vi "Output Complete.vi"(8 "error in  2":errorcluster, 11 "TeleOp Data Cluster 2":T1) -> (0 "error out  2":errorcluster)   [LabVIEW 2018]
uses:
  TypeDefs/Teleop Data Cluster.ctl
  TypeDefs/typedef_enum_Refnums.ctl
  <vilib>/Rock Robotics/WPI/Solenoid/WPI_SolenoidValue.ctl
  <vilib>/Rock Robotics/WPI/ThirdParty/Phoenix-LabVIEW/Motor Controller/Controls/CTRE_Phoenix_MotorControl_ControlMode.ctl
  <vilib>/Rock Robotics/WPI/Solenoid/WPI_SolenoidSetEnum.vi
  <vilib>/Rock Robotics/Network Tables/NT Write Boolean.vi
  <vilib>/Rock Robotics/Network Tables/NT Write Number.vi
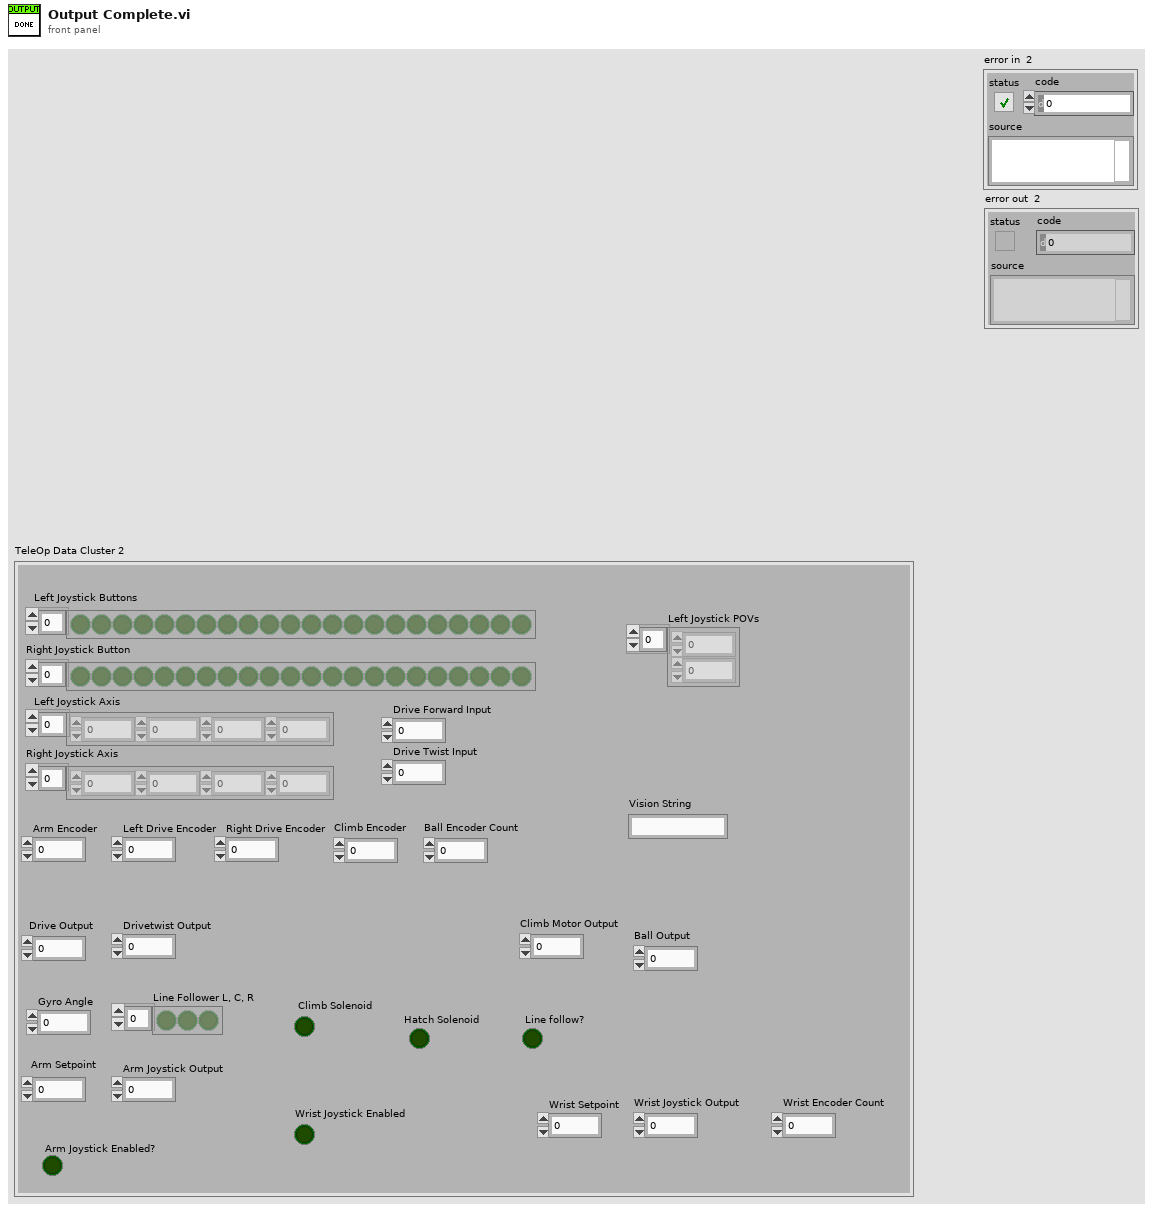
[diagram p1: front panel]
types:
  T1 = typedef "Teleop Data Cluster.ctl" = cluster{"Drive Forward Input ":dbl, "Drive Twist Input":dbl, "Drive Output":dbl, "Drivetwist Output":dbl, "Left Joystick Buttons":bool[], "Left Joystick Axis":dbl[], "Right Joystick Axis":dbl[], "Right Joystick Button":bool[], "Arm Encoder":dbl, "Left Drive Encoder":dbl, "Right Drive Encoder":dbl, "Gyro Angle ":dbl, "Arm Joystick Output  ":dbl, "Line Follower L, C, R ":bool[], "Line follow?":bool, " Climb Solenoid":bool, "Wrist Encoder Count":dbl, "Wrist Joystick Output":dbl, "Ball Encoder Count":dbl, "Ball Output":dbl, "Climb Encoder":dbl, "Climb Motor Output":dbl, " Hatch Solenoid":bool, "Arm Setpoint ":dbl, "Wrist Setpoint ":dbl, "Arm Joystick Enabled?":bool, "Wrist Joystick Enabled":bool, "Vision String":string, "Left Joystick POVs":i16[]}
  T2 = typedef "typedef_enum_Refnums.ctl" = enum16{"Ball_Encoder", "Ball_Motor", "Camera", "Linefollow_3", "Linefollow_2", "Linefollow_1", "Gyro", "Hatch_Solenoid", "Climb_Back_Solenoid", "Arm_Encoder", "Arm_Motor", "Lift_Encoder", "Drive", "Drive_Motor_R", "Drive_Motor_L", "Drive_Encoder_R", "Drive_Encoder_L", "Joy_R", "Joy_L", "Wrist_Motor", "Wrist_Encoder", "Climb Upper Limit", "Climb Lower Limit ", "Climb_Front_Motor"}
  T3 = typedef "CTRE_Phoenix_MotorControl_ControlMode.ctl" = u16
  T4 = typedef "WPI_SolenoidValue.ctl" = enum16{"Off", "On", "Forward", "Reverse"}
  T5 = typedef "WPI_SwitchDevRef.ctl" = cluster{"DevStatus":errorcluster, "DIO Channel":T6, "CntIndex":T7, "Normally Closed":bool}
  T6 = typedef "FPGA_DIOChannel.ctl" = enum8{"DIO 0", "DIO 1", "DIO 2", "DIO 3", "DIO 4", "DIO 5", "DIO 6", "DIO 7", "DIO 8", "DIO 9", "DIO MXP 0", "DIO MXP 1", "DIO MXP 2", "DIO MXP 3", "DIO MXP 4", "DIO MXP 5", "DIO MXP 6", "DIO MXP 7", "DIO MXP 8", "DIO MXP 9", "DIO MXP 10", "DIO MXP 11", "DIO MXP 12", "DIO MXP 13", "DIO MXP 14", "DIO MXP 15", "SPI Port CS1", "SPI Port CS2", "SPI Port CS3", "SPI Port MISO", "SPI Port MOSI", "Invalid"}
  T7 = typedef "FPGA_CounterCtrSystemIndex.ctl" = enum8{"Ctr 0", "Ctr 1", "Ctr 2", "Ctr 3", "Ctr 4", "Ctr 5", "Ctr 6", "Ctr 7", "Invalid"}
  T8 = typedef "WPI_MotorControlDeviceRef.ctl" = cluster{"DeviceStatus":errorcluster, "Type":T9, "PWM":cluster{"PWM Channel":T10, "DeadBand":T11}, "CAN":cluster{"Device Number":u8, "SetOutput VI Ref":variant, "GetOutput VI Ref":variant, "Enable VI Ref":variant, "Disable VI Ref":variant, "Data":variant}, "Invert":bool, "DIO PWM":cluster{"PWM \"Enable\" Channel":T10, "DIOChannel":T6, "PWM Rate":dbl}}
  T9 = typedef "WPI_MotorControlType.ctl" = enum16{"PWM", "CAN", "DIO PWM"}
  T10 = typedef "FPGA_DIOPWMChannel.ctl" = enum8{"PWM 0", "PWM 1", "PWM 2", "PWM 3", "PWM 4", "PWM 5", "PWM 6", "PWM 7", "PWM 8", "PWM 9", "PWM MXP 0", "PWM MXP 1", "PWM MXP 2", "PWM MXP 3", "PWM MXP 4", "PWM MXP 5", "PWM MXP 6", "PWM MXP 7", "PWM MXP 8", "PWM MXP 9", "Invalid"}
  T11 = typedef "WPI_PWMDeadband.ctl" = cluster{"Name":string, "maxPositivePwm":i32, "minPositivePwm":i32, "centerPwm":i32, "maxNegativePwm":i32, "minNegativePwm":i32, "angularRange":u16}
  T12 = typedef "WPI_SolenoidDevRef.ctl" = cluster{"DevStatus":errorcluster, "Pneumatics Control Module":u8, "Forward Solenoid Channel":T13, "Reverse Solenoid Channel":T13}
  T13 = typedef "WPI_SolenoidChannel.ctl" = enum8{"Solenoid 0", "Solenoid 1", "Solenoid 2", "Solenoid 3", "Solenoid 4", "Solenoid 5", "Solenoid 6", "Solenoid 7", "Invalid"}
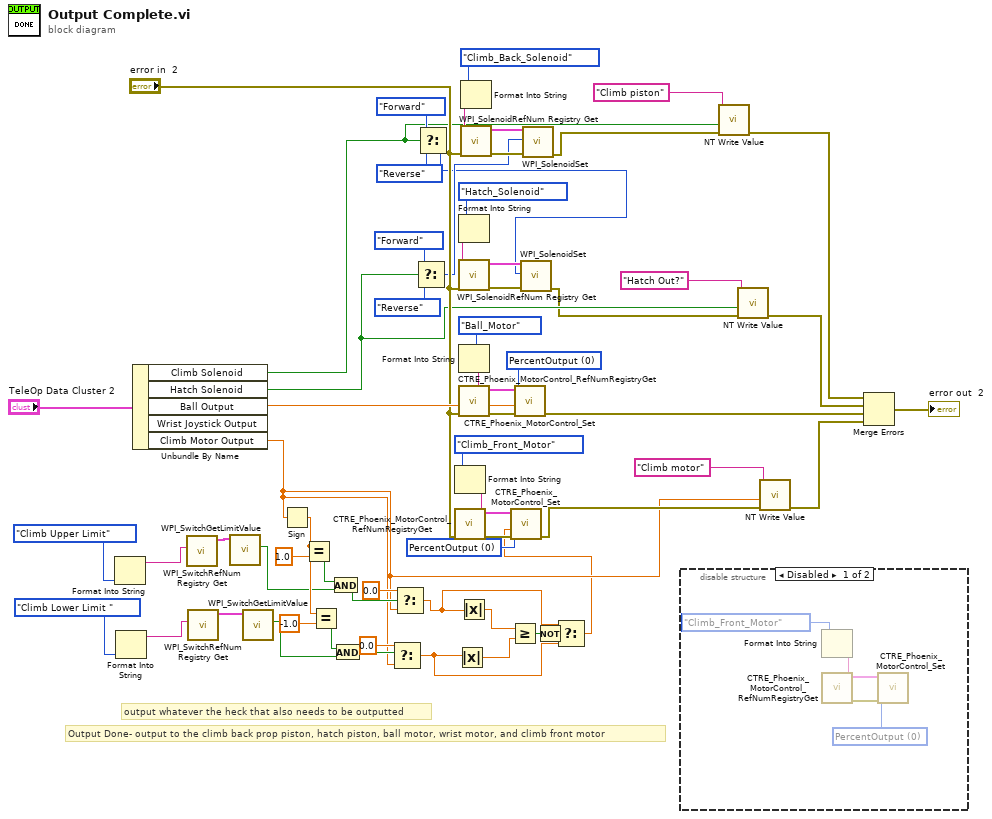
[diagram p0: block diagram]
diagram:
  w40 = T3 0 items=["PercentOutput"=0, "Position"=1, "Velocity"=2, "Current"=3, "Follower"=5, "MotionProfile"=6, "MotionMagic"=7, "MotionProfileArc"=10, "Disabled"=15] ("Control Mode")
  w41 = T3 0 items=["PercentOutput"=0, "Position"=1, "Velocity"=2, "Current"=3, "Follower"=5, "MotionProfile"=6, "MotionMagic"=7, "MotionProfileArc"=10, "Disabled"=15] ("Control Mode")
  # "Output Done- output to the climb back prop piston, hatch piston, ball motor, wrist motor, and climb front motor"
  # "output whatever the heck that also needs to be outputted"
  n1 = Format Into String(typedef_enum_Refnums."Climb Upper Limit" ("RefNums")) -> (resulting string=w26:string)  [unwired: 3 in, 1 out]
  n2 = Format Into String(typedef_enum_Refnums."Climb Lower Limit " ("RefNums")) -> (resulting string=w23:string)  [unwired: 3 in, 1 out]
  n3 = Unbundle By Name("TeleOp Data Cluster 2") -> ("Climb Solenoid"=w35:bool, "Hatch Solenoid"=w36:bool, "Ball Output"=w54:dbl, "Climb Motor Output"=w10:dbl)  [unwired: 1 out]
  n4 = call <vilib>:"WPI_SwitchRefNum Registry Get.vi"("refnum name"=w26) -> ("SwitchDevRef"=w25:T5)  [unwired: 9 in, 1 out]
  n5 = call <vilib>:"WPI_SwitchRefNum Registry Get.vi"("refnum name"=w23) -> ("SwitchDevRef"=w22:T5)  [unwired: 9 in, 1 out]
  n6 = call <vilib>:"WPI_SwitchGetLimitValue.vi"("SwitchDevRef"=w25) -> ("Switch Pressed"=w17:bool)  [unwired: 8 in, 2 out]
  n7 = call <vilib>:"WPI_SwitchGetLimitValue.vi"("SwitchDevRef"=w22) -> ("Switch Pressed"=w15:bool)  [unwired: 8 in, 2 out]
  n8 = Sign(1:w10) -> (0:w19:dbl)
  n9 = Equal?(x=w19, y=1.0) -> (x = y?=w18:bool)
  n10 = Equal?(x=w19, y=-1.0) -> (x = y?=w16:bool)
  n11 = And(x=w18, y=w17) -> (x .and. y?=w14:bool)
  n12 = And(x=w16, y=w15) -> (x .and. y?=w11:bool)
  n13 = Select(t=0.0, s=w11, f=w10) -> (s? t:f=w5:dbl)
  n14 = Select(t=0.0, s=w14, f=w10) -> (s? t:f=w6:dbl)
  n15 = Select(t=WPI_SolenoidValue."Forward" ("Value"), s=w36, f=WPI_SolenoidValue."Reverse" ("Value")) -> (s? t:f=w2:T4)
  n16 = Select(t=WPI_SolenoidValue."Forward" ("Value"), s=w35, f=WPI_SolenoidValue."Reverse" ("Value")) -> (s? t:f=w1:T4)
  n17 = Format Into String(typedef_enum_Refnums."Climb_Front_Motor" ("RefNums")) -> (resulting string=w52:string)  [unwired: 3 in, 1 out]
  n18 = call <vilib>:"CTRE_Phoenix_MotorControl_RefNumRegistryGet.vi"("error in (no error)"="error in  2", "refnum name"=w52) -> ("error out"=w51:errorcluster, "PhoenixMotorControlDevRef"=w50:T8)  [unwired: 8 in]
  n19 = Absolute Value(x=w5) -> (abs(x)=w8:dbl)
  n20 = Format Into String(typedef_enum_Refnums."Hatch_Solenoid" ("RefNums")) -> (resulting string=w63:string)  [unwired: 3 in, 1 out]
  n21 = call <vilib>:"WPI_SolenoidRefNum Registry Get.vi"("error in (no error)"="error in  2", "refnum name"=w63) -> ("error out"=w62:errorcluster, "SolenoidDevRef"=w61:T12)  [unwired: 8 in]
  n22 = Format Into String(typedef_enum_Refnums."Ball_Motor" ("RefNums")) -> (resulting string=w57:string)  [unwired: 3 in, 1 out]
  n23 = call <vilib>:"CTRE_Phoenix_MotorControl_RefNumRegistryGet.vi"("error in (no error)"="error in  2", "refnum name"=w57) -> ("error out"=w56:errorcluster, "PhoenixMotorControlDevRef"=w55:T8)  [unwired: 8 in]
  n24 = Absolute Value(x=w6) -> (abs(x)=w9:dbl)
  n25 = Format Into String(typedef_enum_Refnums."Climb_Back_Solenoid" ("RefNums")) -> (resulting string=w47:string)  [unwired: 3 in, 1 out]
  n26 = call <vilib>:"WPI_SolenoidRefNum Registry Get.vi"("error in (no error)"="error in  2", "refnum name"=w47) -> ("error out"=w46:errorcluster, "SolenoidDevRef"=w45:T12)  [unwired: 8 in]
  n27 = Greater Or Equal?(x=w9, y=w8) -> (x >= y?=w7:bool)
  n28 = call <vilib>:"CTRE_Phoenix_MotorControl_Set.vi"("error in (no error)"=w56, "Output"=w54, "Control Mode"=w41, "PhoenixMotorControlDevRef"=w55) -> ("error out"=w30:errorcluster)  [unwired: 6 in, 1 out]
  n29 = call-poly <vilib>:"WPI_SolenoidSet.vi"("error in (no error)"=w62, "Value"=w1, "SolenoidDevRef"=w61) -> ("error out"=w32:errorcluster)  [unwired: 7 in, 1 out]
  n30 = call-poly <vilib>:"WPI_SolenoidSet.vi"("error in (no error)"=w46, "Value"=w2, "SolenoidDevRef"=w45) -> ("error out"=w34:errorcluster)  [unwired: 7 in, 1 out]
  n31 = Not(x=w7) -> (.not. x?=w3:bool)
  n32 = Select(t=w6, s=w3, f=w5) -> (s? t:f=w4:dbl)
  n33 = call <vilib>:"CTRE_Phoenix_MotorControl_Set.vi"("error in (no error)"=w51, "Output"=w4, "Control Mode"=w40, "PhoenixMotorControlDevRef"=w50) -> ("error out"=w29:errorcluster)  [unwired: 6 in, 1 out]
  n34 = disable-structure shown="Disabled" {
    frame Disabled {
      w66 = T3 0 items=["PercentOutput"=0, "Position"=1, "Velocity"=2, "Current"=3, "Follower"=5, "MotionProfile"=6, "MotionMagic"=7, "MotionProfileArc"=10, "Disabled"=15] ("Control Mode")
      n35 = Format Into String(typedef_enum_Refnums."Climb_Front_Motor" ("RefNums")) -> (resulting string=w69:string)  [unwired: 3 in, 1 out]
      n36 = call <vilib>:"CTRE_Phoenix_MotorControl_RefNumRegistryGet.vi"("refnum name"=w69) -> ("error out"=w68:errorcluster, "PhoenixMotorControlDevRef"=w67:T8)  [unwired: 9 in]
      n37 = call <vilib>:"CTRE_Phoenix_MotorControl_Set.vi"("error in (no error)"=w68, "Control Mode"=w66, "PhoenixMotorControlDevRef"=w67) -> ()  [unwired: 7 in, 2 out]
    }
    frame Enabled {
    }
  }
  n38 = call-poly <vilib>:"NT Write Value.vi"("error in"=w34, "Boolean"=w35, "Name"="Climb piston") -> ("error out"=w33:errorcluster)  [unwired: 8 in]
  n39 = call-poly <vilib>:"NT Write Value.vi"("error in"=w32, "Boolean"=w36, "Name"="Hatch Out?") -> ("error out"=w31:errorcluster)  [unwired: 8 in]
  n40 = call-poly <vilib>:"NT Write Value.vi"("error in"=w29, "Numeric"=w10, "Name"="Climb motor") -> ("error out"=w28:errorcluster)  [unwired: 8 in]
  n41 = Merge Errors(w33, w31, w30, w28) -> (→"error out  2":errorcluster)
